vi "Modbus_Get_Float_Data.vi"(8 "error in (no error)":errorcluster, 10 "Starting Address (2 Bytes)":u16, 11 "TCP Network Connection in":refnum<k5>) -> (0 "error out":errorcluster, 1 "Exception Code":u8 format="%.0x", 2 "Numeric":sgl, 3 "TCP Network Connection out":refnum<k5>)   [LabVIEW 2014]
uses:
  <vilib>/NI Modbus.llb/MB Ethernet Master Query Read Holding Registers (poly).vi
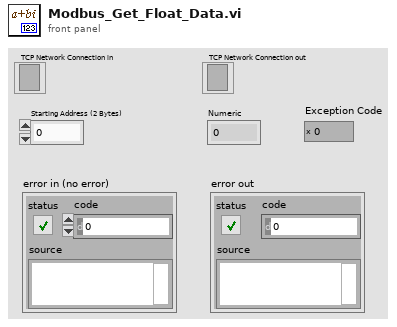
[diagram p1: front panel]
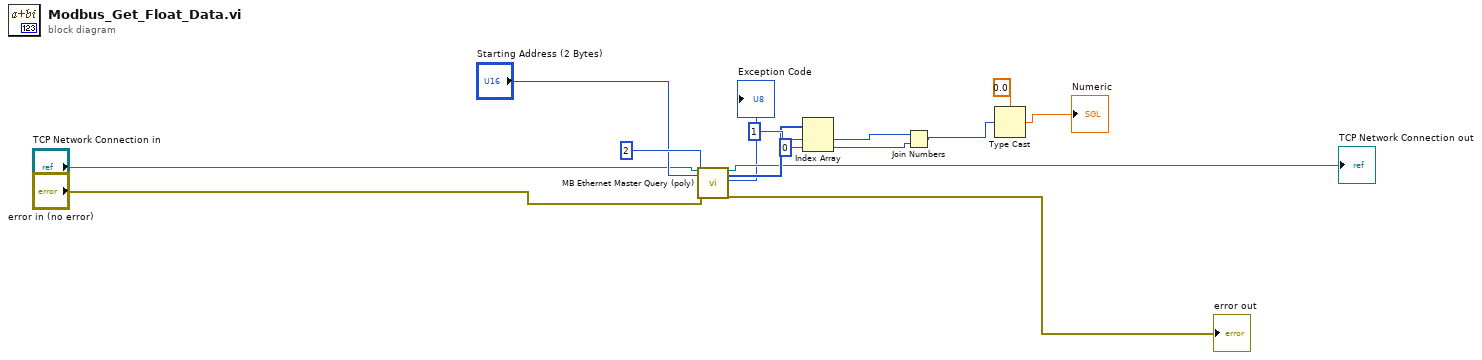
[diagram p0: block diagram]
diagram:
  n1 = call-poly <vilib>:"MB Ethernet Master Query (poly).vi"("TCP Connection Refnum in"="TCP Network Connection in", "Starting Address"="Starting Address (2 Bytes)", "Quantity"=u16 2, "error in"="error in (no error)") -> ("TCP Connection Refnum (dup)"=→"TCP Network Connection out":refnum<k5>, "Holding Registers"=w7:u16[], "Exception Code"=→"Exception Code":u8, "error out"=→"error out":errorcluster)  [unwired: 1 in, 11 out]
  n2 = Index Array(array=w7, index #1=1 ("index"), index #2=0 ("index")) -> (element #1=w10:u16, element #2=w9:u16)
  n3 = Join Numbers(hi=w10, lo=w9) -> ((hi.lo)=w13:u32)
  n4 = Type Cast(type=sgl 0.0, x=w13) -> (*(type *) &x=→"Numeric":sgl)
